vi "Encoder to Distance.vi"(11 "Encoder Value":dbl) -> (3 "Distance (in.)":dbl)   [LabVIEW 2019]
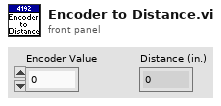
[diagram p1: front panel]
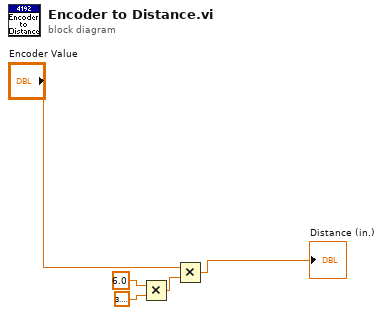
[diagram p0: block diagram]
diagram:
  n1 = Multiply(x=6.0, y=3.141592653589793) -> (x*y=w3:dbl)
  n2 = Multiply(x="Encoder Value", y=w3) -> (x*y=→"Distance (in.)":dbl)
